vi "02 Valves and Power SS.vi"() -> ()   [LabVIEW 2009]
uses:
  <vilib>/DAQmx/write.llb/DAQmx Write (Digital U32 1Chan 1Samp).vi
panel:
  in  "stop":bool
  in  "Valves":bool[](array[boolean])
  in  "Power":bool[](array[boolean])=[TRUE, TRUE, TRUE, TRUE]
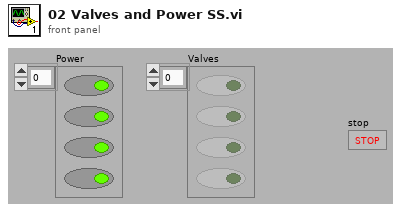
[diagram p1: front panel]
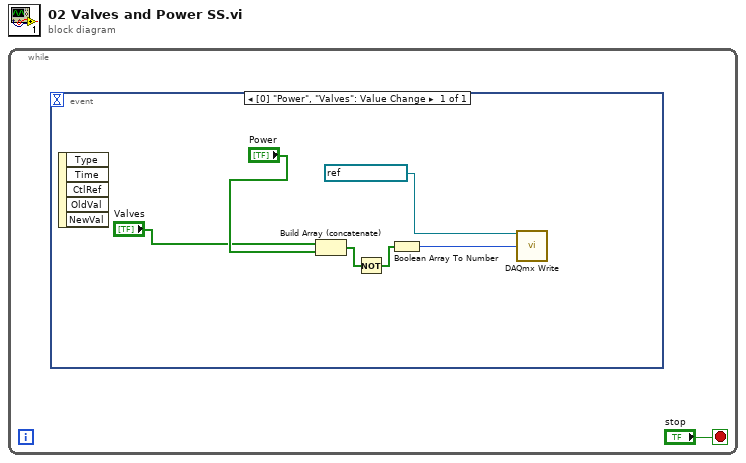
[diagram p0: block diagram]
diagram:
  n1 = while {
    stop <- "stop" stop-if-true
    n2 = event shown="[0] \"Power\", \"Valves\": Value Change" {
      selector: _ -> [_]
      dyn-events: _ -> [_]
      timeout: _ -> [_]
      event [0] "Power", "Valves": Value Change {
        n3 = event-data() -> ()  [unwired: 1 in, 5 out]
        n4 = Build Array (concatenate)("Valves", "Power") -> (w3:bool[])
        n5 = Not(x=w3) -> (.not. x?=w2:bool[])
        n6 = Boolean Array To Number(Boolean array=w2) -> (number=w7:u32)
        n7 = call-poly <vilib>:"DAQmx Write.vi"("task/channels in"=refnum<k21> "SS DO Task", "data"=w7) -> ()  [unwired: 11 in, 3 out]
      }
    }
  }
